vi "Sweep channel.vi"(8 "Error In":errorcluster, 10 "Sweep settings":T1={"Channel to sweep"=0, "Vstart"=0.0, "Vstop"=0.0, "Vstep"=0.0125, "Time interval"=10, "All other chans value"=0.0} {"All other chans value" min=0 max=204.8 step=0.0125 format="%#_g V"; "Time interval" min=10 max=20000 step=5 format="%.0f ms"; "Vstep" min=0.0125 max=204.8 step=0.0125 format="%#_g V"; "Vstop" min=0 max=204.8 step=0.0125 format="%#_g V"; "Vstart" min=0 max=204.8 step=0.0125 format="%#_g V"; "Channel to sweep" max=31 step=1}, 11 "Arduino Port":refnum<visa-resource-name>) -> (0 "Error Out":errorcluster, 3 "Arduino Port out":refnum<visa-resource-name>)   [LabVIEW 2016]
doc: "Perform a voltage sweep of the \"channel to sweep\" of the AD5535 from \"Vstart\" to \"Vstop\" with \"Vstep\" resolution. \n\"Time interval\" defines the step time. \"All other chans value\" set the voltage value of all the other channels of the AD5535 before the sweep is started."
uses:
  Typedef/AD5535 - Sweep settings.ctl
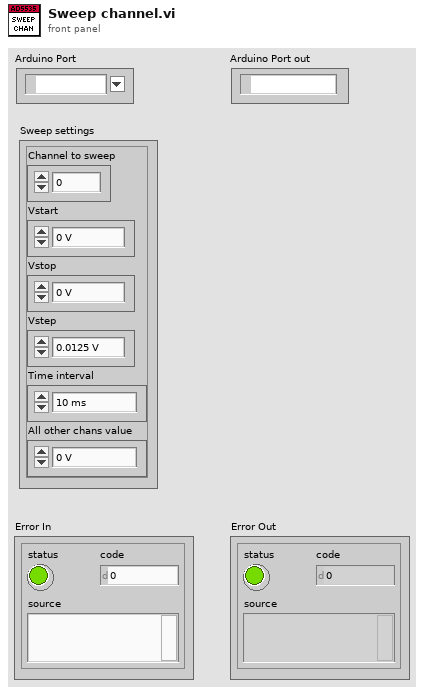
[diagram p1: front panel]
types:
  T1 = typedef "AD5535 - Sweep settings.ctl" = cluster{"Channel to sweep":u8, "Vstart":sgl, "Vstop":sgl, "Vstep":sgl, "Time interval":u32, "All other chans value":sgl}
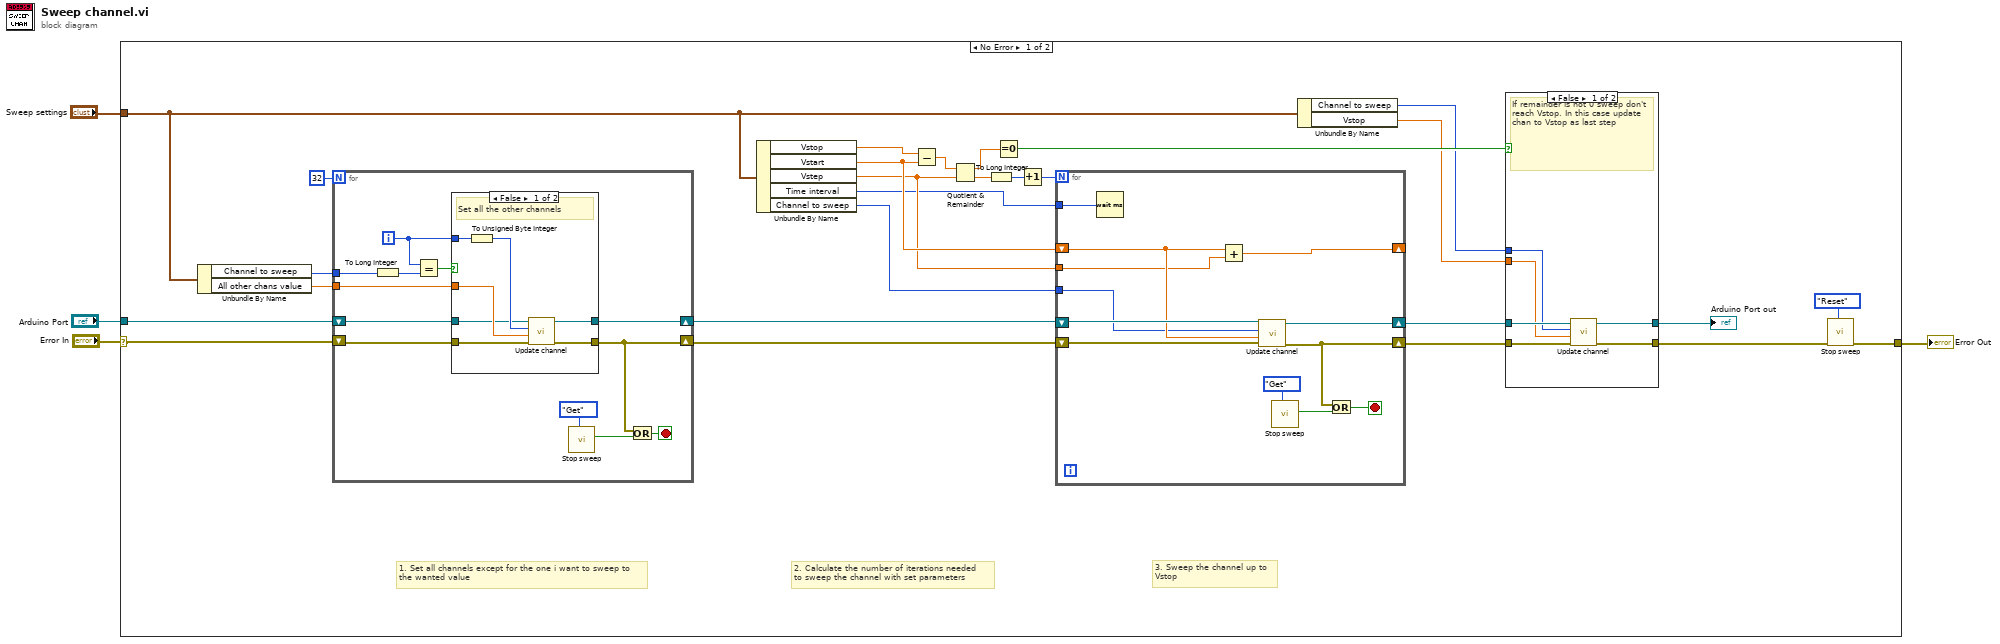
[diagram p0: block diagram]
diagram:
  n1 = case shown="No Error" "Error In" {
    selector: "Error In" -> [w16 w73]
    tunnel: "Arduino Port" -> [w28 _]
    tunnel: "Sweep settings" -> [w7 _]
    tunnel: [w14 w73] -> w2
    frame No Error {
      # "3. Sweep the channel up to\nVstop"
      # "2. Calculate the number of iterations needed\nto sweep the channel with set parameters"
      # "1. Set all channels except for the one i want to sweep to\nthe wanted value"
      n2 = Unbundle By Name(w7) -> ("Channel to sweep"=w30:u8, "All other chans value"=w31:sgl)
      n3 = for {
        N: 32 -> [_]
        tunnel: w31 -> [w63]
        tunnel: w30 -> [w60]
        shift-right: [w56] -> w24
        shift-left: w28 -> [w58]
        shift-right: [w54] -> w23
        shift-left: w16 -> [w57]
        i -> [w59]
        stop <- w55 stop-if-true
        n4 = To Long Integer(number=w60) -> (32bit integer=w61:i32)
        n5 = Equal?(x=w59, y=w61) -> (x = y?=w62:bool)
        n6 = case shown="False" w62 {
          tunnel: w63 -> [w70 _]
          tunnel: w59 -> [w69 _]
          tunnel: w58 -> [w67 w72]
          tunnel: w57 -> [w66 w71]
          tunnel: [w65 w72] -> w56
          tunnel: [w64 w71] -> w54
          frame False {
            # "Set all the other channels"
            n7 = To Unsigned Byte Integer(number=w69) -> (unsigned 8bit integer=w68:u8)
            n8 = call "Update channel.vi"("Error In"=w66, "Value"=w70, "Channel"=w68, "Arduino Port"=w67) -> ("Error Out"=w64:errorcluster, "Arduino Port out"=w65:refnum<visa-resource-name>)  [unwired: 6 in]
          }
          frame True {
            # "Don't send data to the channel to sweep"
          }
        }
        n9 = call "Stop sweep.vi"("Status"=enum16{"Set", "Get", "Reset"}."Get") -> ("Exit?"=w53:bool)  [unwired: 9 in, 1 out]
        n10 = Or(x=w54, y=w53) -> (x .or. y?=w55:bool)
      }
      n11 = Unbundle By Name(w7) -> ("Vstop"=w27:sgl, "Vstart"=w22:sgl, "Vstep"=w21:sgl, "Time interval"=w20:u32, "Channel to sweep"=w19:u8)
      n12 = Subtract(x=w27, y=w22) -> (x-y=w26:sgl)
      n13 = Quotient & Remainder(x=w26, y=w21) -> (x-y*floor(x/y)=w13:sgl, floor(x/y)=w25:sgl)
      n14 = To Long Integer(number=w25) -> (32bit integer=w18:i32)
      n15 = Equal To 0?(x=w13) -> (x = 0?=w12:bool)
      n16 = Increment(x=w18) -> (x+1=w17:i32)
      n17 = for {
        N: w17 -> [_]
        shift-right: [w40] -> w10
        shift-left: w23 -> [w50]
        shift-right: [w49] -> w11
        shift-left: w24 -> [w51]
        tunnel: w21 -> [w47]
        shift-right: [w46] -> _
        shift-left: w22 -> [w48]
        tunnel: w20 -> [w45]
        tunnel: w19 -> [w44]
        stop <- w41 stop-if-true
        n18 = Wait (ms)(milliseconds to wait=w45) -> ()  [unwired: 1 out]
        n19 = Add(x=w48, y=w47) -> (x+y=w46:sgl)
        n20 = call "Update channel.vi"("Error In"=w50, "Value"=w48, "Channel"=w44, "Arduino Port"=w51) -> ("Error Out"=w40:errorcluster, "Arduino Port out"=w49:refnum<visa-resource-name>)  [unwired: 6 in]
        n21 = call "Stop sweep.vi"("Status"=enum16{"Set", "Get", "Reset"}."Get") -> ("Exit?"=w43:bool)  [unwired: 9 in, 1 out]
        n22 = Or(x=w40, y=w43) -> (x .or. y?=w41:bool)
      }
      n23 = Unbundle By Name(w7) -> ("Channel to sweep"=w6:u8, "Vstop"=w5:sgl)
      n24 = case shown="False" w12 {
        tunnel: w11 -> [w37 w38]
        tunnel: w10 -> [w36 w39]
        tunnel: [w35 w39] -> w9
        tunnel: [w34 w38] -> w8
        tunnel: w6 -> [w33 _]
        tunnel: w5 -> [w32 _]
        frame False {
          # "If remainder is not 0 sweep don't reach Vstop. In this case update chan to Vstop as last step"
          n25 = call "Update channel.vi"("Error In"=w36, "Value"=w32, "Channel"=w33, "Arduino Port"=w37) -> ("Error Out"=w35:errorcluster, "Arduino Port out"=w34:refnum<visa-resource-name>)  [unwired: 6 in]
        }
        frame True {
        }
      }
      "Arduino Port out" <- w8
      n26 = call "Stop sweep.vi"("Status"=enum16{"Set", "Get", "Reset"}."Reset", "Error In"=w9) -> ("Error Out"=w14:errorcluster)  [unwired: 8 in, 1 out]
    }
    frame Error {
    }
  }
  "Error Out" <- w2
